vi "Grabbed data in a VI v4.vi"(11 "[I16] Source Graph\n(samples added to reach 320000)":i16[](graph)=array[320000 elements]) -> ()   [LabVIEW 2020]
uses:
  <vilib>/measure/matone.llb/Extract Multiple Tone Information 1 Chan.vi
  <vilib>/Platform/NI_3dgraph.lvlib
  <vilib>/measure/NI_MAPro.lvlib
panel:
  in  "[I16] Data Graph":i16[](graph)=array[393212 elements]
  in  "number":dbl=200.0
  in  "old keller":bool
  out "Period (ns)":sgl format="%#_6f"
  out "Number of points":i32
  out "DAQ Sampling Period (ns)":sgl format="%#_6f"
  in  "DAQ Sampling Rate (MHz)":sgl=800.0 format="%^#_6g"
  in  "Sliders auto scale":bool=TRUE
  in  "scaling by :200":bool=TRUE
  in  "Laser Frequency (MHz)":dbl=80.2
  in  "Dwell time (ns)":i32=40
  in  "use FT":bool=TRUE
  in  "Absolute value":bool
  in  "Tab Control":T1(tab)
  out "Invalid setup":bool
  in  "Z-Axis Max":dbl(slide)=108704.0 scale=3.0..84921.0 scale format="%#_6f"
  out "max value":i32
  out "min value":i32
  in  "Z-Axis Min":dbl(slide)=2000.0 scale=3.0..84921.0 scale format="%#_6f"
  out "Intensity Graph (manual scaling of Z-axis)":i32[][](graph)
  out "Image":T2(plugin-control)
  in  "Image 1LUT":cluster{dbl, dbl}(slide)={0.0, 32956.62953995158} scale=3.0..84921.0 scale format="%#_10f"
  out "Intensity Graph (autoscaling Z-axis)":i32[][](graph)
  in  "Frame Size":u16(ring)=100 caption="Frame Size\n(ensure this matches \nthe actual size)" items=["20X20"=0, "100X100"=100, "128X128"=128, "200X200"=200, "256X256"=256, "512X512"=512]
  in  "Mode":T3(ring)
  in  "3D graph":refnum<k7>(container)
  out "multiple tone information":T4(array[cluster])=[{"detected frequency"=59.40457132494078, "detected amplitude"=677.5224683183739, "detected phase (deg)"=-6.85916777032908}, {"detected frequency"=10023.302847711435, "detected amplitude"=302.0949374874943, "detected phase (deg)"=265.4481634375171}, {"detected frequency"=20019.602268100927, "detected amplitude"=136.99007273675608, "detected phase (deg)"=123.98051462950585}, {"detected frequency"=30006.01918128676, "detected amplitude"=20.477000538882503, "detected phase (deg)"=-16.173557072223005}] {"detected phase (deg)" format="%_6g"; "detected amplitude" format="%_6p"; "detected frequency" format="%_6p"}
  in  "dt of the data which is analysed":dbl=1.25 format="%#_6f"
  in  "max num tones":i32=5
  out "Number of points":i32
  out "calculated  k":dbl=3.208
  out "cosine":i16[](array[numeric])=[71, 0, -71, -100, -71, 0, 71, 100, 71, 0, -71, -100, -71, 0, 71, 100, 71, 0, -71, -100, -71, 0, 71, 100, 71, 0, -71, -100, -71, 0, 71, 100]
  out "sine":i16[](array[numeric])=[71, 100, 71, 0, -71, -100, -71, 0, 71, 100, 71, 0, -71, -100, -71, 0, 71, 100, 71, 0, -71, -100, -71, 0, 71, 100, 71, 0, -71, -100, -71, 0]
  out "[I32] Processed Data Graph":i32[](graph)
  # "50ns missing points"
  # "4095"
  # "32767"
  # "Only I16 data appears to allow manual z-axis scaling of the image.\n\nHowever when FT is used the data intensities require higher than 16bit resolution. When displaying that data in the \"GrayScale I16\" image the data gets clipped.\n\nWe need to think of a solution if we are going to have to use the VISION image display.\n\nOn the other hand the native LabVIEW intensity graph (blue data)  works fine.\n\nThe output of the FT seems \"crispier\"."
  # "<-- Set this correctly"
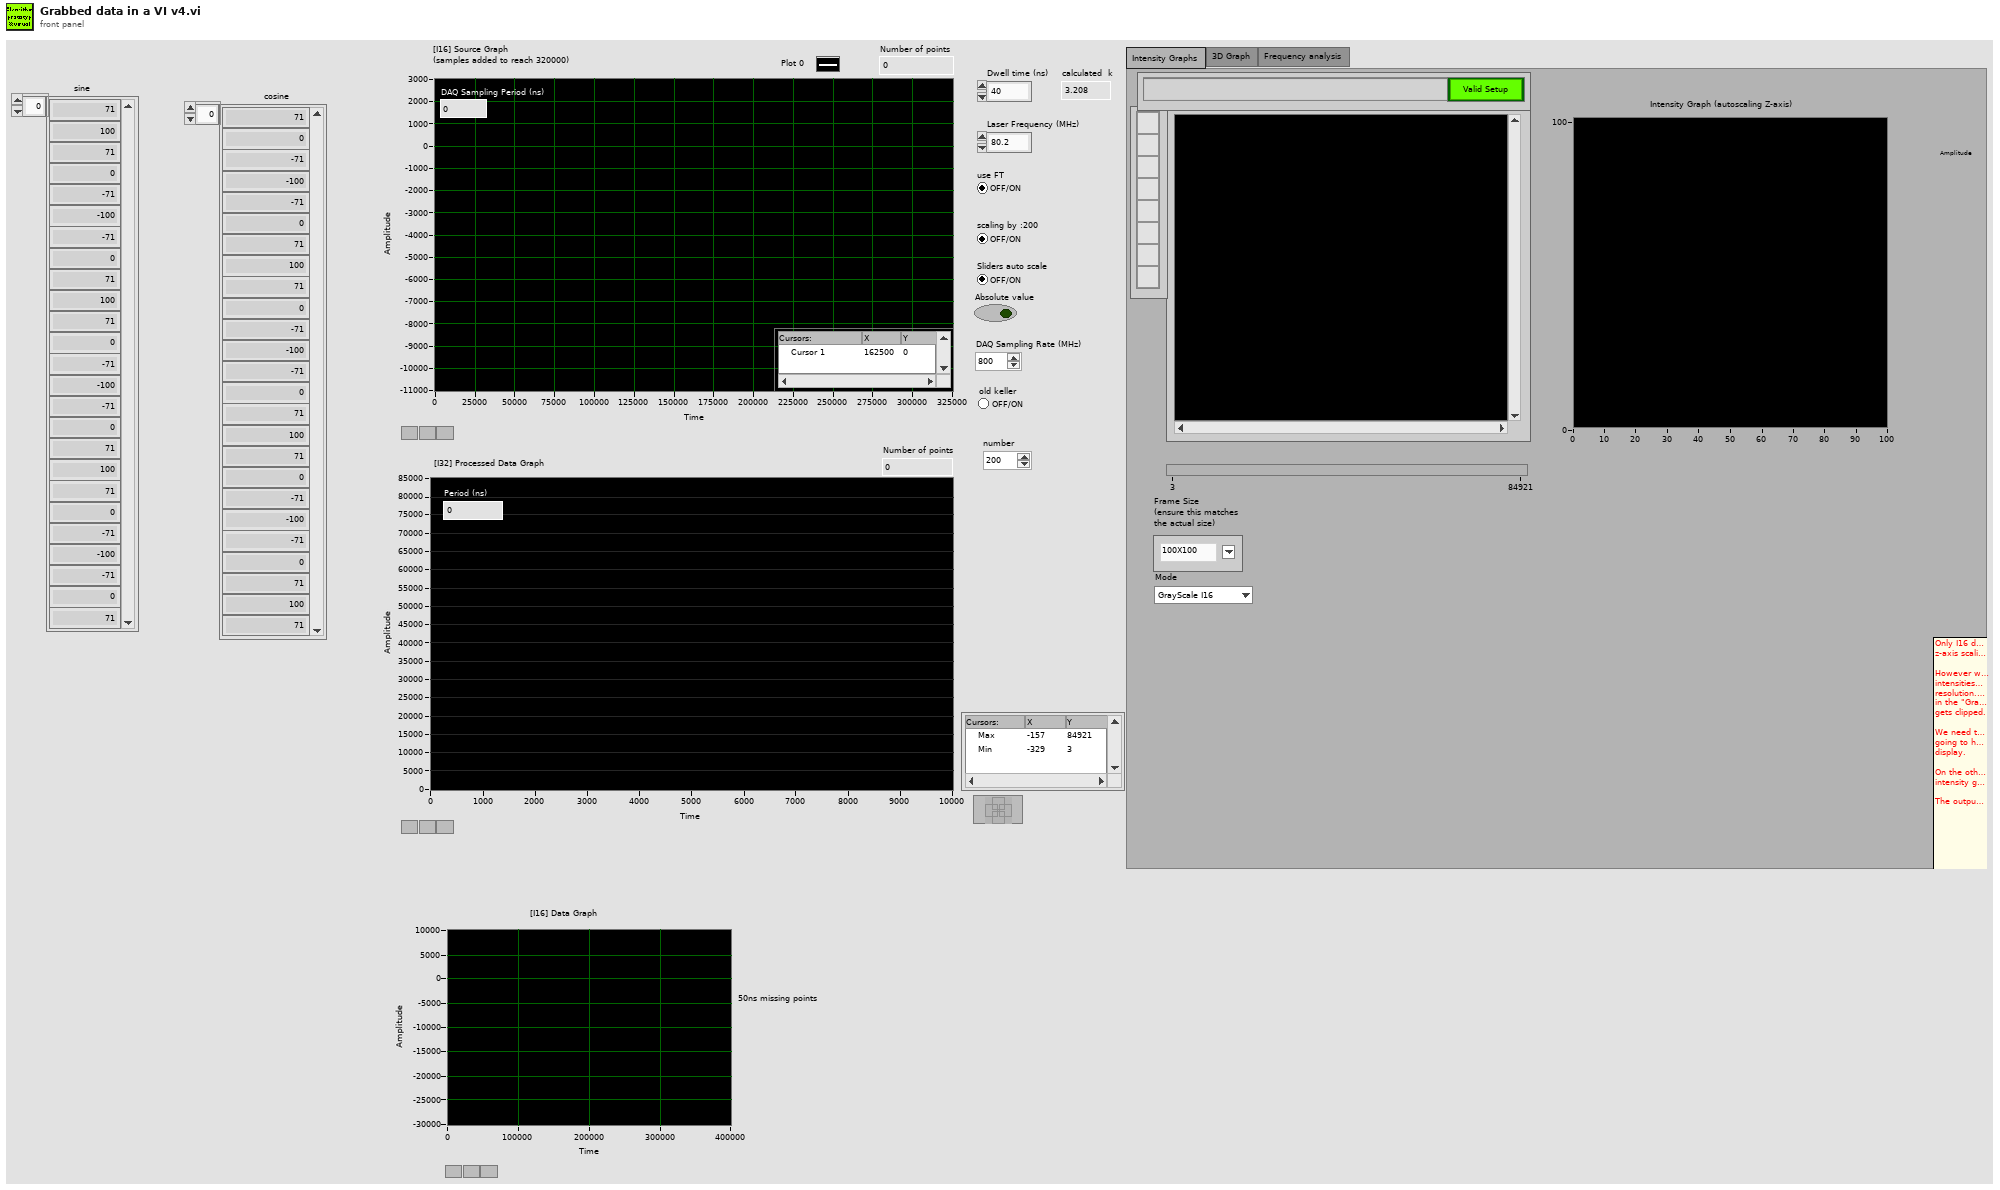
[diagram p1: front panel]
types:
  T1 = enum32{"Intensity Graphs", "3D Graph", "Frequency analysis"}
  T2 = typedef "IMAQ Image.ctl" = refnum<image>
  T3 = enum16{"GrayScale I16", "GrayScale SGL", "Colour U32"}
  T4 = cluster{"detected frequency":dbl, "detected amplitude":dbl, "detected phase (deg)":dbl}[]
  T5 = enum32{"none", "input signal", "detected signal", "residual signal"}
  T6 = cluster{"Conversion Method":u32, "Minimum Value":i32, "Maximum Value":i32, "Number Of Shifts":i32}
  T7 = typedef "Image Type" = u32
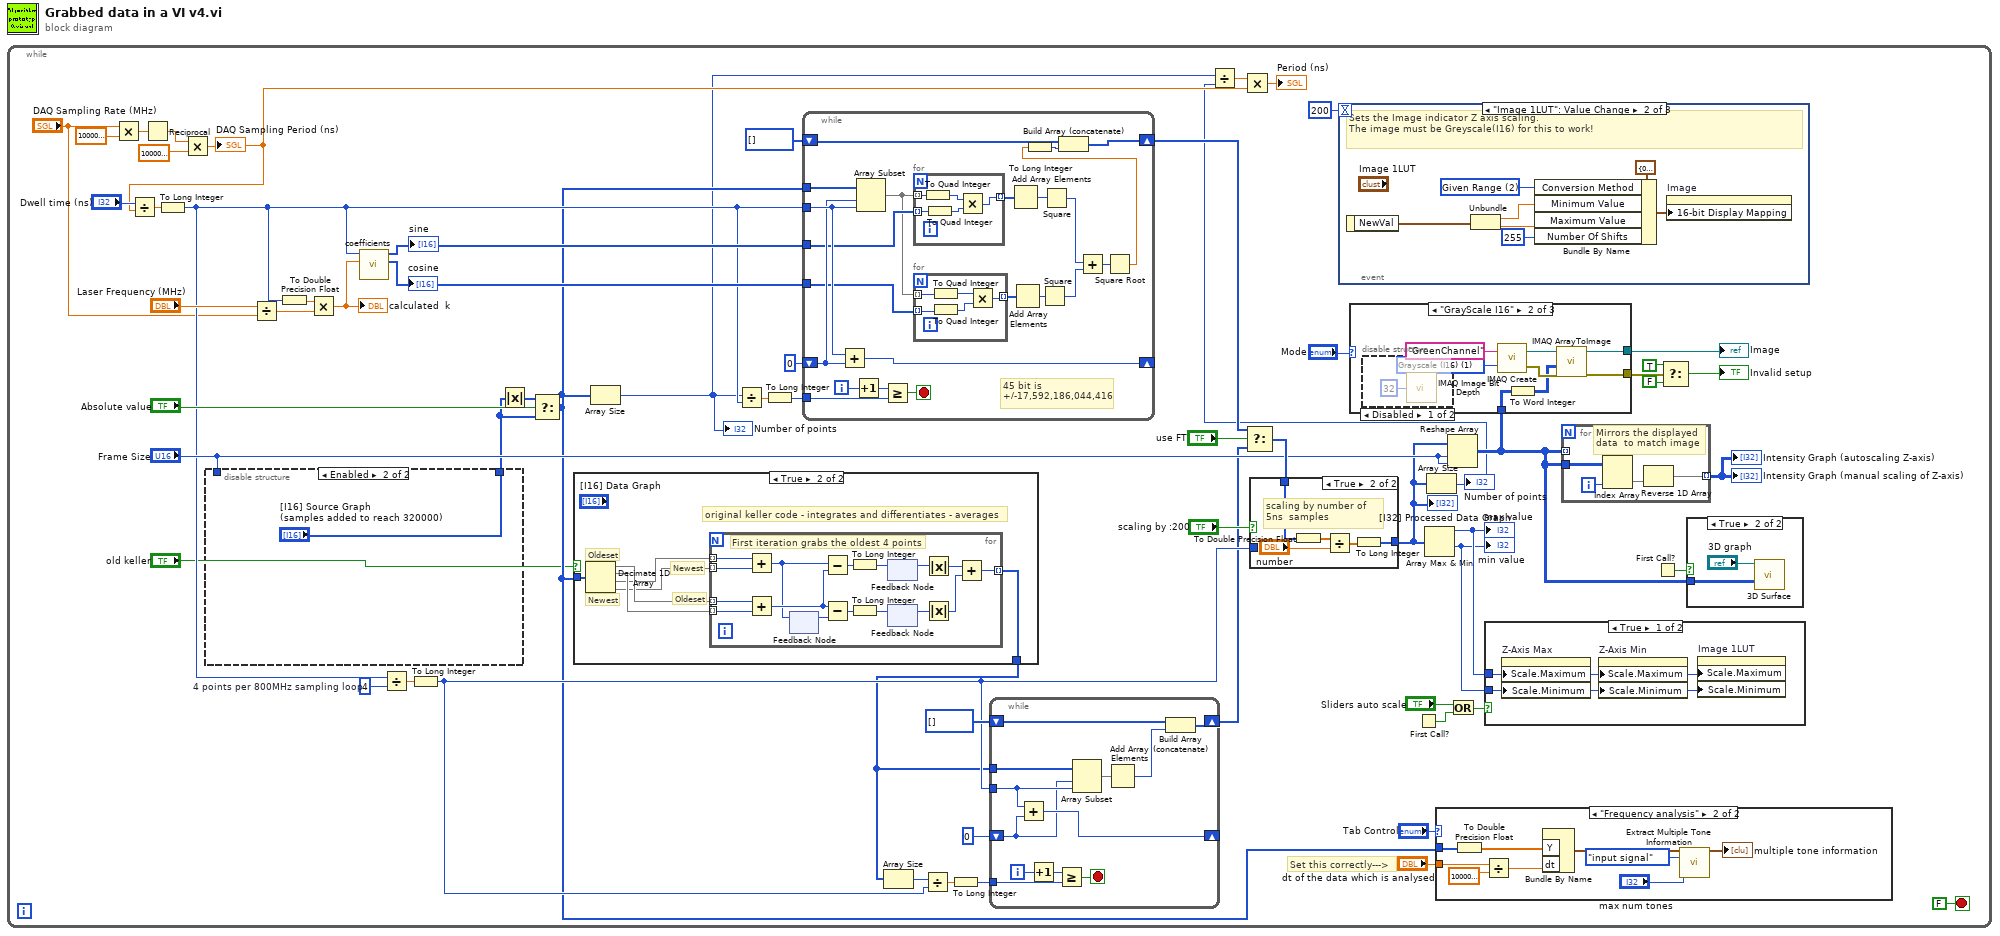
[diagram p0: block diagram]
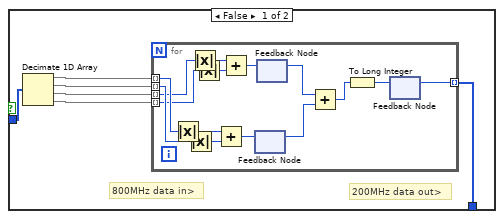
[diagram p2: hidden frame]
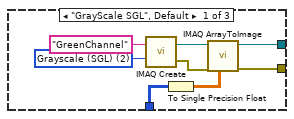
[diagram p5: hidden frame]
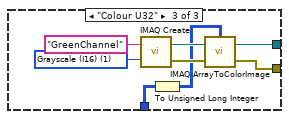
[diagram p7: hidden frame]
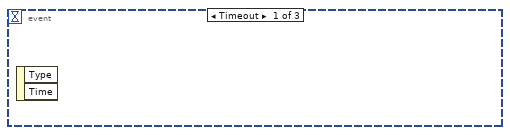
[diagram p8: hidden frame]
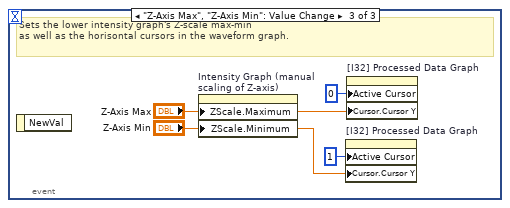
[diagram p9: hidden frame]
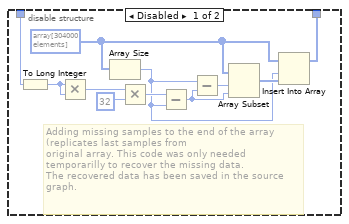
[diagram p10: hidden frame]
diagram:
  n1 = while {
    stop <- FALSE stop-if-true
    w45 = 4  # 4 points per 800MHz sampling loop
    # "Set this correctly--->"
    n2 = Multiply(x="DAQ Sampling Rate (MHz)", y=sgl 1000000.0) -> (x*y=w14:sgl)
    n3 = Reciprocal(x=w14) -> (1/x=w12:sgl)
    n4 = Multiply(x=w12, y=sgl 1000000000.0) -> (x*y=w6:sgl)
    "DAQ Sampling Period (ns)" <- w6
    n5 = Divide(x="Dwell time (ns)", y=w6) -> (x/y=w46:sgl)
    n6 = To Long Integer(number=w46) -> (32bit integer=w34:i32)
    n7 = disable-structure shown="Enabled" {
      disable-tunnel: "Frame Size" -> [w159 _]
      disable-tunnel: [w157 "[I16] Source Graph\n(samples added to reach 320000)"] -> w36
      frame Disabled {
        w158 = i16[] array[304000 elements] ("[I16] Data Graph")
        # "Adding missing samples to the end of the array (replicates last samples from \noriginal array. This code was only needed temporarilly to recover the missing data.\nThe recovered data has been saved in the source graph."
        n8 = To Long Integer(number=w159) -> (32bit integer=w165:i32)
        n9 = Multiply(x=w165, y=w165) -> (x*y=w167:i32)
        n10 = Array Size(array=w158) -> (size(s)=w160:i32)
        n11 = Multiply(x=w167, y=32) -> (x*y=w164:i32)
        n12 = Subtract(x=w164, y=w160) -> (x-y=w163:i32)
        n13 = Subtract(x=w160, y=w163) -> (x-y=w162:i32)
        n14 = Array Subset(array=w158, index=w162, length=w163) -> (w161:i16[])
        n15 = Insert Into Array(array=w158, index=w160, new element=w161) -> (w157:i16[])
      }
      frame Enabled {
      }
    }
    n16 = Divide(x="Laser Frequency (MHz)", y="DAQ Sampling Rate (MHz)") -> (x/y=w33:dbl)
    n17 = To Double Precision Float(number=w34) -> (double precision float=w32:dbl)
    n18 = Multiply(x=w32, y=w33) -> (x*y=w42:dbl)
    "calculated  k" <- w42
    n19 = call "coefficients.vi"("k-constant"=w42, "Numeric"=w34) -> ("cosine"=w49:i16[], "sine"=w50:i16[])  [unwired: 8 in]
    "sine" <- w50
    "cosine" <- w49
    n20 = Divide(x=w34, y=w45) -> (x/y=w44:dbl)
    n21 = To Long Integer(number=w44) -> (32bit integer=w41:i32)
    n22 = Absolute Value(x=w36) -> (abs(x)=w60:i16[])
    n23 = Select(t=w60, s="Absolute value", f=w36) -> (s? t:f=w4:i16[])
    n24 = case shown="True" "old keller" {
      tunnel: [w63 w85] -> w19
      tunnel: w4 -> [w64 w84]
      frame False {
        # "200MHz data out>"
        # "800MHz data in>"
        n25 = Decimate 1D Array(w64) -> (w68:i16[], w67:i16[], w66:i16[], w65:i16[])
        n26 = for {
          tunnel: w68 -> [w80] mode=indexing
          tunnel: w67 -> [w81] mode=indexing
          tunnel: w66 -> [w78] mode=indexing
          tunnel: w65 -> [w79] mode=indexing
          tunnel: [w69] -> w63 mode=indexing
          n27 = Absolute Value(x=w80) -> (abs(x)=w71:i16)
          n28 = Absolute Value(x=w81) -> (abs(x)=w70:i16)
          n29 = Absolute Value(x=w78) -> (abs(x)=w73:i16)
          n30 = Absolute Value(x=w79) -> (abs(x)=w72:i16)
          n31 = Add(x=w71, y=w70) -> (x+y=w77:i16)
          n32 = Add(x=w73, y=w72) -> (x+y=w82:i16)
          n33 = feedback #1() -> (w74:i16)  [unwired: 1 in]
          n34 = feedback-in #1(w77) -> ()
          n35 = feedback #2() -> (w76:i16)  [unwired: 1 in]
          n36 = feedback-in #2(w82) -> ()
          n37 = Add(x=w76, y=w74) -> (x+y=w75:i16)
          n38 = To Long Integer(number=w75) -> (32bit integer=w83:i32)
          n39 = feedback #3() -> (w69:i32)  [unwired: 1 in]
          n40 = feedback-in #3(w83) -> ()
        }
      }
      frame True {
        # "Oldeset"
        # "Newest"
        # "Oldeset"
        # "Newest"
        # "original keller code - integrates and differentiates - averages"
        n41 = Decimate 1D Array(w84) -> (w89:i16[], w88:i16[], w87:i16[], w86:i16[])
        n42 = for {
          tunnel: w89 -> [w92] mode=indexing
          tunnel: w88 -> [w93] mode=indexing
          tunnel: w87 -> [w90] mode=indexing
          tunnel: w86 -> [w91] mode=indexing
          tunnel: [w94] -> w85 mode=indexing
          # "First iteration grabs the oldest 4 points"
          n43 = Add(x=w90, y=w91) -> (x+y=w95:i16)
          n44 = Add(x=w92, y=w93) -> (x+y=w104:i16)
          n45 = feedback #4() -> (w105:i16)  [unwired: 1 in]
          n46 = feedback-in #4(w95) -> ()
          n47 = Subtract(x=w95, y=w104) -> (x-y=w99:i16)
          n48 = Subtract(x=w104, y=w105) -> (x-y=w97:i16)
          n49 = To Long Integer(number=w99) -> (32bit integer=w98:i32)
          n50 = To Long Integer(number=w97) -> (32bit integer=w96:i32)
          n51 = feedback #5() -> (w103:i32)  [unwired: 1 in]
          n52 = feedback-in #5(w98) -> ()
          n53 = feedback #6() -> (w102:i32)  [unwired: 1 in]
          n54 = feedback-in #6(w96) -> ()
          n55 = Absolute Value(x=w103) -> (abs(x)=w101:i32)
          n56 = Absolute Value(x=w102) -> (abs(x)=w100:i32)
          n57 = Add(x=w101, y=w100) -> (x+y=w94:i32)
        }
      }
    }
    n58 = Array Size(array=w4) -> (size(s)=w3:i32)
    "Number of points" <- w3
    n59 = Divide(x=w3, y=w34) -> (x/y=w52:dbl)
    n60 = To Long Integer(number=w52) -> (32bit integer=w51:i32)
    n61 = while {
      tunnel: w4 -> [w198]
      tunnel: w34 -> [w197]
      shift-right: [w196] -> _
      shift-left: 0 -> [w195]
      shift-right: [w194] -> w48
      shift-left: i32[] [] -> [w193]
      tunnel: w51 -> [w191]
      tunnel: w50 -> [w188]
      tunnel: w49 -> [w185]
      i -> [w192]
      stop <- w190 stop-if-true
      # "45 bit is\n+/-17,592,186,044,416"
      n62 = Add(x=w197, y=w195) -> (x+y=w196:i32)
      n63 = Increment(x=w192) -> (x+1=w189:i32)
      n64 = Array Subset "Array Subset"(array=w198, index=w195, length=w197) -> (w186:i16[])
      n65 = Greater Or Equal?(x=w189, y=w191) -> (x >= y?=w190:bool)
      n66 = for {
        tunnel: w186 -> [w208] mode=indexing
        tunnel: w188 -> [w207] mode=indexing
        tunnel: [w206] -> w187 mode=indexing
        n67 = To Quad Integer(1:w208) -> (0:w205:i64)
        n68 = To Quad Integer(1:w207) -> (0:w204:i64)
        n69 = Multiply(x=w205, y=w204) -> (x*y=w206:i64)
      }
      n70 = for {
        tunnel: w186 -> [w203] mode=indexing
        tunnel: w185 -> [w202] mode=indexing
        tunnel: [w201] -> w184 mode=indexing
        n71 = To Quad Integer(1:w203) -> (0:w200:i64)
        n72 = To Quad Integer(1:w202) -> (0:w199:i64)
        n73 = Multiply(x=w200, y=w199) -> (x*y=w201:i64)
      }
      n74 = Add Array Elements(numeric array=w187) -> (sum=w182:i64)
      n75 = Add Array Elements(numeric array=w184) -> (sum=w180:i64)
      n76 = Square(x=w180) -> (x^2=w179:i64)
      n77 = Square(x=w182) -> (x^2=w181:i64)
      n78 = Add(x=w181, y=w179) -> (x+y=w183:i64)
      n79 = Square Root(x=w183) -> (sqrt(x)=w178:dbl)
      n80 = To Long Integer(number=w178) -> (32bit integer=w177:i32)
      n81 = Build Array (concatenate)(w193, w177) -> (w194:i32[])
    }
    n82 = Array Size(array=w19) -> (size(s)=w57:i32)
    n83 = Divide(x=w57, y=w41) -> (x/y=w56:dbl)
    n84 = To Long Integer(number=w56) -> (32bit integer=w55:i32)
    n85 = while {
      tunnel: w19 -> [w220]
      tunnel: w41 -> [w219]
      shift-right: [w218] -> _
      shift-left: 0 -> [w217]
      shift-right: [w214] -> w9
      shift-left: i32[] [] -> [w213]
      tunnel: w55 -> [w211]
      i -> [w212]
      stop <- w210 stop-if-true
      n86 = Add(x=w219, y=w217) -> (x+y=w218:i32)
      n87 = Increment(x=w212) -> (x+1=w209:i32)
      n88 = Greater Or Equal?(x=w209, y=w211) -> (x >= y?=w210:bool)
      n89 = Array Subset "Array Subset"(array=w220, index=w217, length=w219) -> (w216:i32[])
      n90 = Add Array Elements(numeric array=w216) -> (sum=w215:i32)
      n91 = Build Array (concatenate)(w213, w215) -> (w214:i32[])
    }
    n92 = Select(t=w48, s="use FT", f=w9) -> (s? t:f=w38:i32[])
    n93 = case shown="True" "scaling by :200" {
      tunnel: w41 -> [_ _]
      tunnel: w38 -> [w171 w176]
      tunnel: [w171 w175] -> w5
      frame False {
      }
      frame True {
        # "scaling by number of  5ns  samples"
        n94 = To Double Precision Float(number=w176) -> (double precision float=w173:dbl[])
        n95 = Divide(x=w173, y="number") -> (x/y=w174:dbl[])
        n96 = To Long Integer(number=w174) -> (32bit integer=w175:i32[])
      }
    }
    "[I32] Processed Data Graph" <- w5
    n97 = event shown="[1] \"Image 1LUT\": Value Change" {
      selector: _ -> [_ _ _]
      dyn-events: _ -> [_ _ _]
      timeout: 200 -> [_ _ _]
      event Timeout {
        n98 = event-data() -> ()  [unwired: 1 in, 2 out]
      }
      event "Image 1LUT": Value Change {
        w147 = u32 2 items=["Full Dynamic", "Downshift", "Given Range", "90% Dynamic", "Given Percent Range"] ("16-bit Display Mapping:Conversion Method")
        # "Sets the Image indicator Z axis scaling.\nThe image must be Greyscale(I16) for this to work!"
        n99 = event-data() -> ("NewVal"=w146:cluster{dbl, dbl})  [unwired: 1 in]
        n100 = Unbundle(w146) -> (w149:dbl, w148:dbl)
        n101 = Bundle By Name(cluster=T6 {"Conversion Method"=0, "Minimum Value"=0, "Maximum Value"=0, "Number Of Shifts"=0} ("16-bit Display Mapping:All Elements"), "Conversion Method"=w147, "Minimum Value"=w149, "Maximum Value"=w148, "Number Of Shifts"=255) -> (w151:T6)
        n102 = property on="Image" class="ImageControl"("16-bit Display Mapping"=w151) -> ()  [unwired: 2 in, 2 out]
      }
      event "Z-Axis Max", "Z-Axis Min": Value Change {
        # "Sets the lower intensity graph's Z-scale max-min\nas well as the horisontal cursors in the waveform graph."
        n103 = event-data() -> ()  [unwired: 1 in, 1 out]
        n104 = property on="Intensity Graph (manual scaling of Z-axis)" class="IntGraph (strict)"("ZScale.Maximum"="Z-Axis Max", "ZScale.Minimum"="Z-Axis Min") -> ()  [unwired: 2 in, 2 out]
        n105 = property on="[I32] Processed Data Graph" class="WFGraph (strict)"("Active Cursor"=u32 1, "Cursor.Cursor Y"="Z-Axis Min") -> ()  [unwired: 2 in, 2 out]
        n106 = property on="[I32] Processed Data Graph" class="WFGraph (strict)"("Active Cursor"=u32 0, "Cursor.Cursor Y"="Z-Axis Max") -> ()  [unwired: 2 in, 2 out]
      }
    }
    n107 = First Call?() -> (First Call?: T/F=w24:bool)
    n108 = Array Max & Min(array=w5) -> (max value=w31:i32, min value=w30:i32)  [unwired: 2 out]
    "max value" <- w31
    "min value" <- w30
    n109 = Array Size(array=w5) -> (size(s)=w2:i32)
    "Number of points" <- w2
    n110 = Divide(x=w3, y=w2) -> (x/y=w8:dbl)
    n111 = Multiply(x=w8, y=w6) -> (x*y=→"Period (ns)":dbl)
    n112 = case shown="\"Frequency analysis\"" "Tab Control" {
      tunnel: "dt of the data which is analysed" -> [_ w108]
      tunnel: w4 -> [_ w109]
      frame Default {
      }
      frame "Frequency analysis" {
        n113 = To Double Precision Float(number=w109) -> (double precision float=w110:dbl[])
        n114 = Divide(x=w108, y=1000000000.0) -> (x/y=w106:dbl)
        n115 = Bundle By Name("Y"=w110, "dt"=w106) -> (w111:waveform(dbl))  [unwired: 1 in]
        n116 = call-poly <vilib>:"Extract Multiple Tone Information.vi"("time signal in"=w111, "export mode"=T5."input signal", "max num tones"="max num tones") -> ("multiple tone information"=→"multiple tone information":T4)  [unwired: 10 in, 2 out]
      }
    }
    n117 = Reshape Array(w5, "Frame Size", "Frame Size") -> (w21:i32[][])
    n118 = case shown="\"GrayScale I16\"" "Mode" {
      tunnel: [w128 w136 w141] -> w39
      tunnel: w21 -> [w127 w135 w145]
      tunnel: [w126 w134 w140] -> w29
      frame "GrayScale SGL", Default {
        w124 = T7 2 items=["Grayscale (U8)", "Grayscale (I16)", "Grayscale (SGL)", "Complex (CSG)", "RGB (U32)", "HSL (U32)", "RGB (U64)", "Grayscale (U16)"] ("Image Type")
        n119 = call "IMAQ Create"("Image Name"="GreenChannel", "Image Type"=w124) -> ("New Image"=w123:T2, "error out"=w122:errorcluster)  [unwired: 3 in]
        n120 = To Single Precision Float(number=w127) -> (single precision float=w121:sgl[][])
        n121 = call "IMAQ ArrayToImage"("Image Pixels (Float)"=w121, "error in (no error)"=w122, "Image"=w123) -> ("error out"=w126:errorcluster, "Image Out"=w128:T2)  [unwired: 7 in]
      }
      frame "GrayScale I16" {
        w132 = T7 1 items=["Grayscale (U8)", "Grayscale (I16)", "Grayscale (SGL)", "Complex (CSG)", "RGB (U32)", "HSL (U32)", "RGB (U64)", "Grayscale (U16)"] ("Image Type")
        n122 = disable-structure shown="Disabled" {
          frame Disabled {
            n123 = call "IMAQ Image Bit Depth"("Bit Depth (0)"=u32 32) -> ()  [unwired: 12 in, 3 out]
          }
          frame Enabled {
          }
        }
        n124 = call "IMAQ Create"("Image Name"="GreenChannel", "Image Type"=w132) -> ("New Image"=w131:T2, "error out"=w130:errorcluster)  [unwired: 3 in]
        n125 = To Word Integer(number=w135) -> (16bit integer=w129:i16[][])
        n126 = call "IMAQ ArrayToImage"("error in (no error)"=w130, "Image Pixels (I16)"=w129, "Image"=w131) -> ("error out"=w134:errorcluster, "Image Out"=w136:T2)  [unwired: 7 in]
      }
      frame "Colour U32" {
        w143 = T7 1 items=["Grayscale (U8)", "Grayscale (I16)", "Grayscale (SGL)", "Complex (CSG)", "RGB (U32)", "HSL (U32)", "RGB (U64)", "Grayscale (U16)"] ("Image Type")
        n127 = call "IMAQ Create"("Image Name"="GreenChannel", "Image Type"=w143) -> ("New Image"=w142:T2, "error out"=w139:errorcluster)  [unwired: 3 in]
        n128 = To Unsigned Long Integer(number=w145) -> (unsigned 32bit integer=w138:u32[][])
        n129 = call "IMAQ ArrayToColorImage"("Image Pixels (U32)"=w138, "Image"=w142, "error in (no error)"=w139) -> ("Image Out"=w141:T2, "error out"=w140:errorcluster)  [unwired: 2 in]
      }
    }
    "Image" <- w39
    n130 = Or(x="Sliders auto scale", y=w24) -> (x .or. y?=w22:bool)
    n131 = case shown="True" w22 {
      tunnel: w31 -> [w170 _]
      tunnel: w30 -> [w169 _]
      frame True {
        n132 = property on="Z-Axis Max" class="Slide (strict)"("Scale.Maximum"=w170, "Scale.Minimum"=w169) -> ()  [unwired: 2 in, 2 out]
        n133 = property on="Z-Axis Min" class="Slide (strict)"("Scale.Maximum"=w170, "Scale.Minimum"=w169) -> ()  [unwired: 2 in, 2 out]
        n134 = property on="Image 1LUT" class="Slide (strict)"("Scale.Maximum"=w170, "Scale.Minimum"=w169) -> ()  [unwired: 2 in, 2 out]
      }
      frame False {
      }
    }
    n135 = for {
      tunnel: w21 -> [_] mode=indexing
      tunnel: [w120] -> w16 mode=indexing
      tunnel: w21 -> [w119]
      i -> [w118]
      # "Mirrors the displayed\ndata  to match image"
      n136 = Index Array(array=w119, index (col)=w118) -> (element=w117:i32[])  [unwired: 1 in]
      n137 = Reverse 1D Array(array=w117) -> (reversed array=w120:i32[])
    }
    "Intensity Graph (autoscaling Z-axis)" <- w16
    "Intensity Graph (manual scaling of Z-axis)" <- w16
    n138 = First Call?() -> (First Call?: T/F=w20:bool)
    n139 = Select(t=TRUE, s=w29, f=FALSE) -> (s? t:f=→"Invalid setup":bool)
    n140 = case shown="True" w20 {
      tunnel: w21 -> [_ w115]
      frame False {
      }
      frame True {
        n141 = call <vilib>:"3D Surface.vi"("z matrix"=w115, "3D graph"="3D graph") -> ()  [unwired: 8 in, 2 out]
      }
    }
  }
